vi "Construct.vi"(8 "error in":errorcluster, 9 "status error channel data references":T2 {"specific errors"."timeout" format="%.0x"; "specific errors"."bit timing" format="%.0x"; "specific errors"."long word" format="%.0x"; "specific errors"."parity" format="%.0x"; "specific errors"."gap" format="%.0x"; "receiving" format="%.0x"}, 10 "RT hardware channels":T3[](array[typedef]) {"labels settings for RT"."Label Timestamp Channel Data Reference" format="%.0x"; "labels settings for RT"."Word Initial Raw Value" format="%032.0f"; "labels settings for RT"."Label Disable/Trigger Channel Reference" format="%.0x"; "labels settings for RT"."parameter driver data"."Tx parameter refs" format="%.0x"; "labels settings for RT"."SDI" format="%02b"; "labels settings for RT"."label" format="%.0o"}, 11 "ID":string) -> (0 "error out":errorcluster, 3 "AIM ARINC-429 Rx execution unit":refnum<class "Rx Execution Unit.lvclass">)   [LabVIEW 2020, in "AIM ARINC 429 Engine.lvlib" / "Implementation.lvlib" / "Rx Execution Unit.lvclass"]
uses:
  Rx Execution Unit.lvclass
  Shared/Label.ctl
  <vilib>/NI/NI VeriStand Encoding and Decoding/Encoding.ctl
  <vilib>/NI/NI VeriStand Encoding and Decoding/Encoding and Decoding.lvlib
  Shared/Parameter Definition.ctl
  <vilib>/NI VeriStand/Custom Device API/Data Reference.ctl
  <vilib>/NI VeriStand/Custom Device API/Custom Device API.lvlib
  <vilib>/NI VeriStand/Custom Device API/Custom Device Item Ref.ctl
  Shared/RT Parameters.ctl
  Shared/Transfer Type.ctl
  Shared/RT Label Settings.ctl
  Shared/RT Hardware Channel Settings.ctl
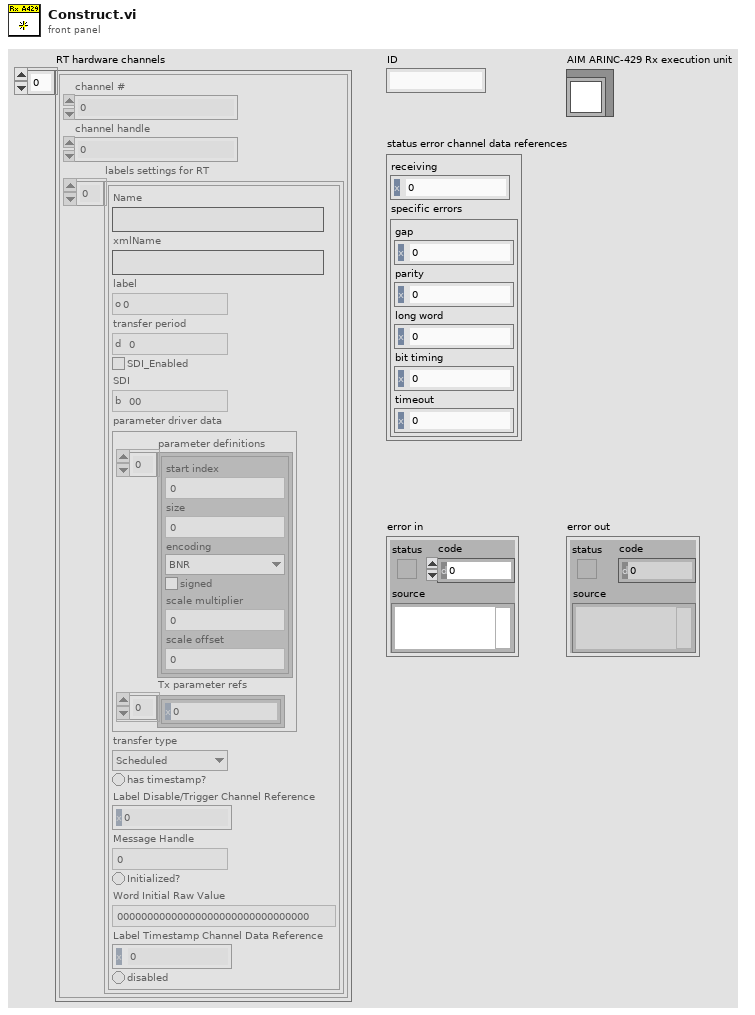
[diagram p1: front panel]
types:
  T1 = typedef "Custom Device API.lvlib/Data Reference.ctl" = i32
  T2 = cluster{"receiving":T1, "specific errors":cluster{"gap":T1, "parity":T1, "long word ":T1, "bit timing":T1, "timeout":T1}}
  T3 = typedef "RT Hardware Channel Settings.ctl" = cluster{"channel #":u16, "channel handle":u64, "labels settings for RT":T4[]}
  T4 = typedef "RT Label Settings.ctl" = cluster{"Name":string, "xmlName":string, "label":T5, "transfer period":u32, "SDI_Enabled":bool, "SDI":u8, "parameter driver data":T6, "transfer type":T10, "has timestamp?":bool, "Label Disable/Trigger Channel Reference":T9, "Message Handle":u64, "Initialized?":bool, "Word Initial Raw Value":u32, "Label Timestamp Channel Data Reference":T1, "disabled":bool}
  T5 = typedef "Label.ctl" = u8
  T6 = typedef "RT Parameters.ctl" = cluster{"parameter definitions":T7[], "Tx parameter refs":T9[]}
  T7 = typedef "Parameter Definition.ctl" = cluster{"start index":i32, "size":i32, "encoding":T8, "signed":bool, "scale multiplier":dbl, "scale offset":dbl}
  T8 = typedef "Encoding and Decoding.lvlib/Encoding.ctl" = enum16{"BNR", "BCD", "Discrete"}
  T9 = typedef "Custom Device API.lvlib/Custom Device Item Ref.ctl" = u64
  T10 = typedef "Transfer Type.ctl" = enum16{"Scheduled", "Acyclic", "Block", "Strobe"}
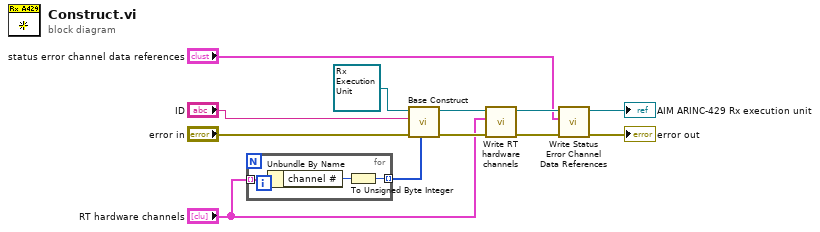
[diagram p0: block diagram]
diagram:
  n1 = for {
    tunnel: "RT hardware channels" -> [w15] mode=indexing
    tunnel: [w13] -> w1 mode=indexing
    n2 = Unbundle By Name(w15) -> ("channel #"=w14:u16)
    n3 = To Unsigned Byte Integer(number=w14) -> (unsigned 8bit integer=w13:u8)
  }
  n4 = call-dynamic "Base Construct.vi"("channels"=w1, "error in"="error in", "identifier"="ID", "execution unit in"=refnum<class "Rx Execution Unit.lvclass"> refnum ("Ballard ARINC-429 Rx Execution Unit in")) -> ("error out"=w5:errorcluster, "execution unit out"=w3:refnum<class "Rx Execution Unit.lvclass">)  [unwired: 6 in]
  n5 = call "Write RT hardware channels.vi"("error in"=w5, "RT hardware channels"="RT hardware channels", "Rx execution unit in"=w3) -> ("error out"=w10:errorcluster, "Rx execution unit out"=w12:refnum<class "Rx Execution Unit.lvclass">)  [unwired: 7 in]
  n6 = call "Write Status Error Channel Data References.vi"("error in"=w10, "status error channel data references"="status error channel data references", "Rx execution unit in"=w12) -> ("error out"=→"error out":errorcluster, "Rx execution unit out"=→"AIM ARINC-429 Rx execution unit":refnum<class "Rx Execution Unit.lvclass">)  [unwired: 7 in]
